vi "Eagle_RT Get Green Cordinates.vi"(8 "error in":errorcluster, 11 "FPGA Reference":T1) -> (0 "error out":errorcluster)   [LabVIEW 2015]
uses:
  Eagle RT FPGA Ref.ctl
  Controls/Eagle Green Cordinates.ctl
  Stream/Controls/RT Streamer State.ctl
  <vilib>/Utility/error.llb/Error Cluster From Error Code.vi
  <vilib>/rvi/errors/niLvFpgaAdjustHostInterfaceError.vi
  <vilib>/rvi/interface/nirviMethod/nirviMethod.xnode
  <vilib>/rvi/interface/nirviMethod/StockFPGA_InlinedMethodWaitForSingleIRQ.vi
  <vilib>/FPGAPlugInAG/Dynamic/niLvFpga_WaitOnIrq_Dynamic.vi
  <vilib>/FPGAPlugInAG/Dynamic/niLvFpga_ReadFifo_Dynamic.vi
  <vilib>/rvi/errors/niLvFpgaMergeErrorWithErrorCode.vi
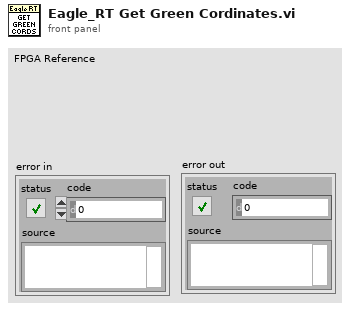
[diagram p1: front panel]
types:
  T1 = typedef "Eagle RT FPGA Ref.ctl" = refnum<k20>
  T2 = typedef "RT Streamer State.ctl" = enum16{"Init", "Idle", "Stream", "Listen", "SetRefrashRate", "SendCmdAck", "SendCmdDone", "SendSysState", "StartRecord", "Green Cordinates", "Error"}
  T3 = typedef "Eagle Green Cordinates.ctl" = cluster{"X Cord":u16[], "Y Cord":u16[]}
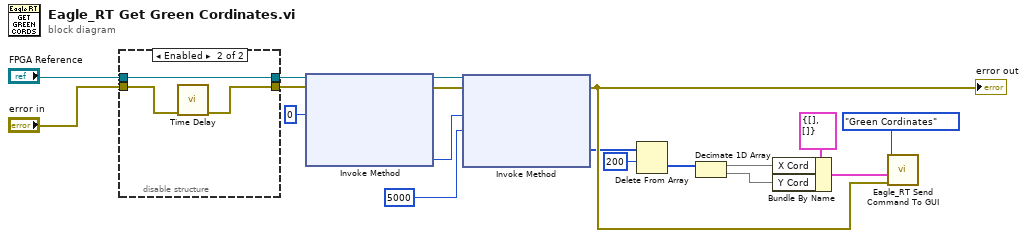
[diagram p0: block diagram]
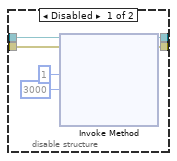
[diagram p2: hidden frame]
diagram:
  n1 = disable-structure shown="Enabled" {
    disable-tunnel: [w24 w26] -> w13
    disable-tunnel: [w23 w25] -> w12
    disable-tunnel: "FPGA Reference" -> [w20 w25]
    disable-tunnel: "error in" -> [w19 w27]
    frame Disabled {
      n2 = xnode "Invoke Method"("FPGA VI Reference In"=w20, "error in"=w19, "IRQ Number(s)"=1, "Timeout (ms)"=3000) -> ("FPGA VI Reference Out"=w23:T1, "error out"=w24:errorcluster)  [unwired: 2 out]
    }
    frame Enabled {
      n3 = call "Time Delay"("error in (no error)"=w27) -> ("error out"=w26:errorcluster)  [unwired: 10 in]
    }
  }
  n4 = xnode "Invoke Method"("FPGA VI Reference In"=w12, "error in"=w13, "Number of Elements"=u32 0) -> ("FPGA VI Reference Out"=w15:T1, "error out"=w16:errorcluster, "Elements Remaining"=w17:u32)  [unwired: 1 in, 1 out]
  n5 = xnode "Invoke Method"("FPGA VI Reference In"=w15, "error in"=w16, "Number of Elements"=w17, "Timeout (ms)"=5000) -> ("error out"=w5:errorcluster, "Data"=w3:u16[])  [unwired: 2 out]
  "error out" <- w5
  n6 = Delete From Array(array=w3, length=200) -> (deleted portion=w1:u16[])  [unwired: 1 in, 1 out]
  n7 = Decimate 1D Array(w1) -> (w9:u16[], w8:u16[])
  n8 = Bundle By Name(cluster=T3 {"X Cord"=[], "Y Cord"=[]}, "X Cord"=w9, "Y Cord"=w8) -> (w7:T3)
  n9 = call "Eagle_RT Send Command To GUI.vi"("Error in"=w5, "Data"=w7, "CMD"=RT_Streamer_State."Green Cordinates") -> ()  [unwired: 8 in, 1 out]
